vi "Temp_QCM_MKS_file.vi"() -> ()   [LabVIEW 2013]
doc: "This example demonstrates temperature control and monitoring.\n\nNote:\nBefore start this VI is it necessary:\n\n- preconfigure some specific parameters that are not supported by this driver (e.g. PV-I/O Type, Linearization type, Alarm Input Values... ) by Quick Codes, or by Eurotherm iTools or by instrument front panel controls\n- enter correct VISA Resource Descriptor, Device Address and Baud Rate into front-panel controls"
uses:
  LabVIEW Drivers for DVS instruments/_mks/common/mks pressure units.ctl
  LabVIEW Drivers for DVS instruments/_mks/common/mks status.ctl
  LabVIEW Drivers for DVS instruments/_mks/common/mks status control mode.ctl
  LabVIEW Drivers for DVS instruments/_mks/common/mks status learning mode.ctl
  LabVIEW Drivers for DVS instruments/_mks/common/mks status selection mode.ctl
  LabVIEW Drivers for DVS instruments/_mks/common/mks control direction.ctl
  LabVIEW Drivers for DVS instruments/_mks/common/mks setup communication mode.ctl
  LabVIEW Drivers for DVS instruments/_mks/common/mks setup termination character.ctl
  LabVIEW Drivers for DVS instruments/_mks/common/mks setpoint type.ctl
  LabVIEW Drivers for DVS instruments/_mks/common/mks control type.ctl
  <vilib>/Utility/file.llb/Write To Spreadsheet File (string).vi
  <instrlib>/Eurotherm 32xx Series/Eurotherm 32xx Series.lvlib
panel:
  in  "stop":bool
  in  "Tab Control":T1(tab)
  in  "Add comments to the data file here and click outside the comment box to submit.\nThe time at which comments are submitted is saved in the data file.":string
  out "New ALARM !":bool
  in  "Acknowledge All Alarms":bool
  in  "Controller  Mode":u8(ring) items=["Auto", "Manual"]
  in  "Temp Setpoint (C)":i16(slide)=25 min=0 max=1300 scale=0.0..500.0
  out "Temperature (C)":sgl
  out "Process Value - Chart":sgl(graph)
  in  "Keylock":u8(ring) items=["None", "All", "Edit", "mod", "mAn", "Stby", "tmr"]
  out "Alarm Output":bool
  in  "Alarm \nNumber (1)":u16=1 min=1 max=4
  out "Freq and Resistance Graph":T2(graph)
  out "pressure units 3":T3
  out "Waveform Chart 2":dbl(graph)
  out "status 2":T4
  out "Pressure 2":dbl
  in  "Control direction 3":T8
  in  "Setpoint 2":dbl(knob) min=0.0 max=100.0 scale=0.0..100.0
  out "Control direction 4":T8
  # "Configuring Instrument\n \nPlease Wait......\n\nChart will update in 20 sec"
  # "Instructions:\n\nMake sure all instruments are plugged into the correct ports, the correct port numbers are set, and all instruments are turned on. \n\nTo begin, click the RUN arrow on the toolbar, and wait 20 seconds for instruments to begin recording.\n\nTo end, click \"END DATA LOGGING\". DO NOT press the STOP button on the toolbar."
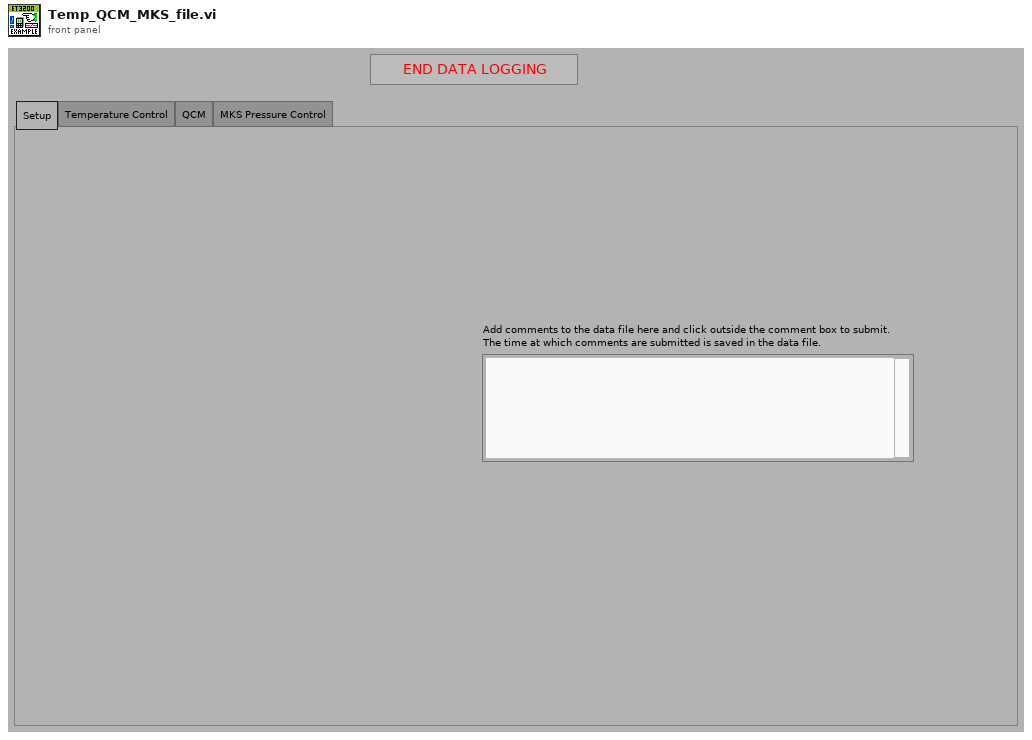
[diagram p1: front panel]
types:
  T1 = enum32{"Setup", "Temperature Control", "QCM", "MKS Pressure Control"}
  T2 = cluster{"XY chart data":cluster{"x":dbl, "y":dbl}[]}[]
  T3 = typedef "mks pressure units.ctl" = enum16{"Torr", "mTorr", "mbar", "ubar", "kPa", "Pa", "cmH2O", "inH2O"}
  T4 = typedef "mks status.ctl" = cluster{"control mode":T5, "learning mode":T6, "selection mode":T7}
  T5 = typedef "mks status control mode.ctl" = enum16{"local", "remote"}
  T6 = typedef "mks status learning mode.ctl" = enum16{"not learning", "learning system", "learning valve"}
  T7 = typedef "mks status selection mode.ctl" = enum16{"open", "close", "stop", "setpoint A", "setpoint B", "setpoint C", "setpoint D", "setpoint E", "analog setpoint"}
  T8 = typedef "mks control direction.ctl" = enum16{"direct", "reverse"}
  T9 = typedef "mks setup termination character.ctl" = enum16{"CRLF", "CR"}
  T10 = typedef "mks setup communication mode.ctl" = enum16{"8 databits no parity", "7 databits even parity"}
  T11 = typedef "mks control type.ctl" = enum16{"Self-Tuning", "PID"}
  T12 = typedef "mks setpoint type.ctl" = enum16{"position", "pressure"}
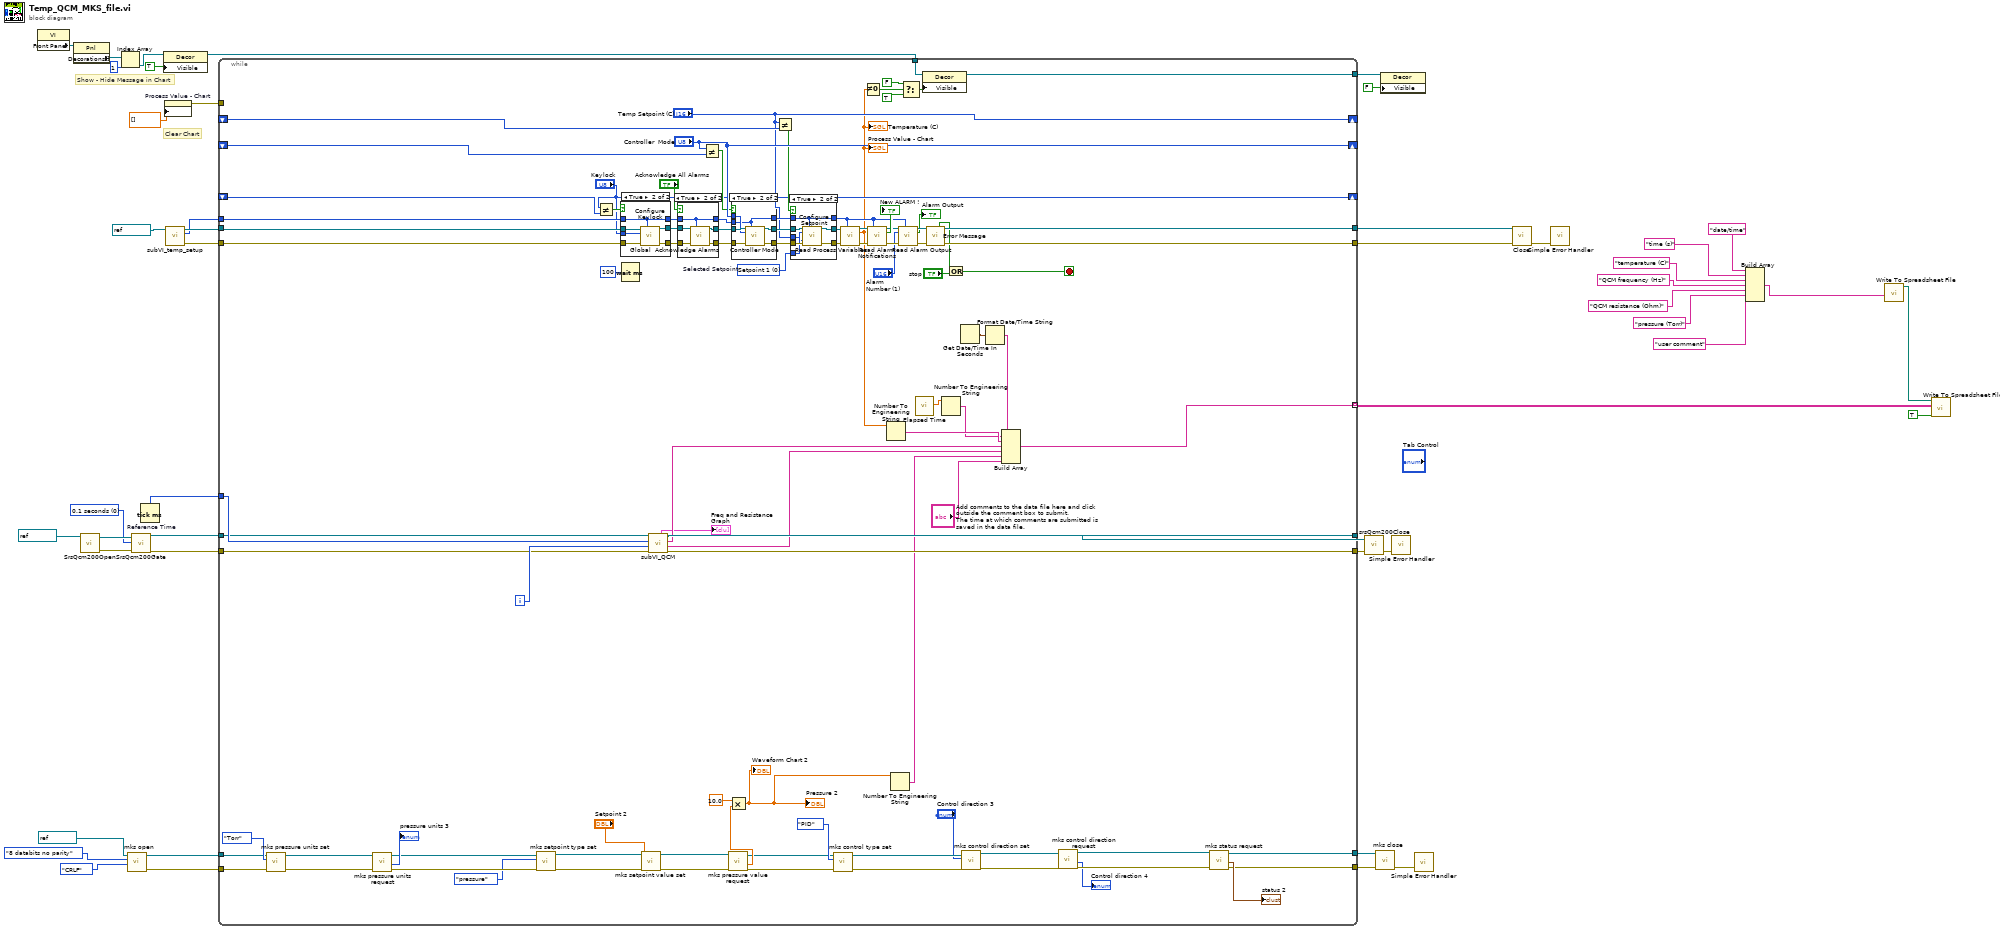
[diagram p0: block diagram]
diagram:
  w21 = u16 0 items=["0.1 seconds", "1.0 seconds", "10.0 seconds"] ("Gate in")
  # "Show - Hide Message in Chart"
  # "Clear Chart"
  n1 = property class="VI"() -> ("Front Panel"=w39:refnum<vi>)  [unwired: 2 in, 2 out]
  n2 = property class="Pnl"(reference=w39) -> ("Decorations[]"=w40:refnum<vi>[])  [unwired: 1 in, 2 out]
  n3 = call <instrlib>:"SrsQcm200Open.vi"("VISA in"=refnum<visa-resource-name> "COM6") -> ("error out"=w25:errorcluster, "VISA out"=w24:refnum<visa-resource-name>)  [unwired: 4 in]
  n4 = Index Array(array=w40, index=1) -> (element=w37:refnum<vi>)
  n5 = call "mks open.vi"("termination character"=mks_setup_termination_character."CRLF", "comm. mode"=mks_setup_communication_mode."8 databits no parity", "VISA in"=refnum<visa-resource-name> "COM5") -> ("error out"=w6:errorcluster, "VISA out"=w7:refnum<visa-resource-name>)  [unwired: 7 in]
  n6 = call <instrlib>:"SrsQcm200Gate.vi"("VISA in"=w24, "Gate in"=w21, "error in (no error)"=w25) -> ("VISA out"=w18:refnum<visa-resource-name>, "error out"=w17:errorcluster)  [unwired: 14 in, 1 out]
  n7 = Tick Count (ms) "Reference Time"() -> (millisecond timer value=w19:u32)
  n8 = property class="Decor"(reference=w37, "Visible"=TRUE) -> (reference out=w36:refnum<vi>)  [unwired: 1 in, 1 out]
  n9 = property on="Process Value - Chart" class="WFChart (strict)"("History Data"=sgl[] []) -> (error out=w32:errorcluster)  [unwired: 2 in, 1 out]
  n10 = call "subVI_temp_setup.vi"("VISA Refnum in"=refnum<visa-resource-name> "COM4" ("VISA resource name")) -> ("error out"=w45:errorcluster, "Unit Address (1)"=w26:u8, "VISA Refnum out"=w46:refnum<visa-resource-name>)  [unwired: 8 in]
  n11 = while {
    tunnel: w46 -> [w113]
    tunnel: w45 -> [w112]
    tunnel: w26 -> [w114]
    tunnel: [w134] -> w43
    tunnel: [w133] -> w44
    shift-right: ["Keylock"] -> _
    shift-left: _ -> [w123]
    shift-right: ["Controller  Mode"] -> _
    shift-left: _ -> [w120]
    shift-right: ["Temp Setpoint (C)"] -> _
    shift-left: _ -> [w118]
    tunnel: w36 -> [w98]
    tunnel: [w96] -> w34
    tunnel: w32 -> [_]
    tunnel: [w92] -> w20 mode=indexing
    tunnel: w19 -> [w90]
    tunnel: w18 -> [w89]
    tunnel: w17 -> [w88]
    tunnel: [w87] -> w16
    tunnel: [w86] -> w15
    tunnel: w7 -> [w56]
    tunnel: w6 -> [w55]
    tunnel: [w54] -> w4
    tunnel: [w53] -> w3
    i -> [w91]
    stop <- w127 stop-if-true
    w129 = u8 0 items=["Setpoint 1", "Setpoint 2", "Alternate Setpoint", "Target Setpoint"]  # Selected Setpoint
    n12 = call "mks pressure units set.vi"("error in (no error)"=w55, "pressure units"=mks_pressure_units."Torr", "VISA in"=w56) -> ("error out"=w69:errorcluster, "VISA out"=w68:refnum<visa-resource-name>)  [unwired: 7 in]
    n13 = call "mks pressure units request.vi"("error in (no error)"=w69, "VISA in"=w68) -> ("error out"=w71:errorcluster, "pressure units"=→"pressure units 3":T3, "VISA out"=w70:refnum<visa-resource-name>)  [unwired: 7 in]
    n14 = call "mks setpoint type set.vi"("error in (no error)"=w71, "setpoint type"=mks_setpoint_type."pressure", "VISA in"=w70) -> ("error out"=w59:errorcluster, "VISA out"=w58:refnum<visa-resource-name>)  [unwired: 7 in]
    n15 = Not Equal?(x="Keylock", y=w123) -> (x != y?=w122:bool)
    n16 = case shown="True" w122 {
      tunnel: w113 -> [w171 w178]
      tunnel: w112 -> [w170 w177]
      tunnel: [w171 w176] -> w142
      tunnel: [w170 w175] -> w141
      tunnel: w114 -> [w172 w174]
      tunnel: [w172 w174] -> w131
      tunnel: "Keylock" -> [_ w173]
      frame False {
      }
      frame True {
        n17 = call <instrlib>:"Configure Keylock.vi"("VISA resource name"=w178, "Unit Address (1)"=w174, "Keylock"=w173, "error in (no error)"=w177) -> ("VISA resource name out"=w176:refnum<visa-resource-name>, "error out"=w175:errorcluster)  [unwired: 10 in]
      }
    }
    n18 = Wait (ms)(milliseconds to wait=u32 100) -> ()  [unwired: 1 out]
    n19 = call "mks setpoint value set.vi"("error in (no error)"=w59, "setpoint"="Setpoint 2", "VISA in"=w58) -> ("error out"=w64:errorcluster, "VISA out"=w63:refnum<visa-resource-name>)  [unwired: 7 in]
    n20 = call "subVI_QCM.vi"("error in (no error)"=w88, "Loop iteration number"=w91, "millisecond timer value"=w90, "VISA Refnum in"=w89) -> ("error out"=w86:errorcluster, "Resistance (Ohm)"=w84:string, "Freq (Hz)"=w85:string, "VISA Refnum out"=w87:refnum<visa-resource-name>, "Freq and Resistance Graph"=→"Freq and Resistance Graph":T2)  [unwired: 3 in]
    n21 = case shown="True" "Acknowledge All Alarms" {
      tunnel: w142 -> [w163 w169]
      tunnel: w141 -> [w162 w168]
      tunnel: [w163 w167] -> w136
      tunnel: [w162 w166] -> w135
      tunnel: w131 -> [w164 w165]
      tunnel: [w164 w165] -> w130
      frame False {
      }
      frame True {
        n22 = call <instrlib>:"Global  Acknowledge Alarms.vi"("VISA resource name"=w169, "Unit Address (1)"=w165, "error in (no error)"=w168) -> ("VISA resource name out"=w167:refnum<visa-resource-name>, "error out"=w166:errorcluster)  [unwired: 11 in]
      }
    }
    n23 = Not Equal?(x="Controller  Mode", y=w120) -> (x != y?=w119:bool)
    n24 = call "mks pressure value request.vi"("error in (no error)"=w64, "VISA in"=w63) -> ("error out"=w66:errorcluster, "pressure"=w81:dbl, "VISA out"=w65:refnum<visa-resource-name>)  [unwired: 7 in]
    n25 = Multiply(x=10.0, y=w81) -> (x*y=w52:dbl)
    "Pressure 2" <- w52
    "Waveform Chart 2" <- w52
    n26 = case shown="True" w119 {
      tunnel: [w153 w161] -> w140
      tunnel: [w154 w160] -> w137
      tunnel: w136 -> [w154 w159]
      tunnel: w135 -> [w153 w158]
      tunnel: w130 -> [w155 w156]
      tunnel: "Controller  Mode" -> [_ w157]
      tunnel: [w155 w156] -> w128
      frame False {
      }
      frame True {
        n27 = call <instrlib>:"Controller Mode.vi"("VISA resource name"=w159, "Unit Address (1)"=w156, "Controller Mode (0: Auto)"=w157, "error in (no error)"=w158) -> ("VISA resource name out"=w160:refnum<visa-resource-name>, "error out"=w161:errorcluster)  [unwired: 10 in]
      }
    }
    n28 = Not Equal?(x="Temp Setpoint (C)", y=w118) -> (x != y?=w116:bool)
    n29 = case shown="True" w116 {
      tunnel: w140 -> [w143 w152]
      tunnel: [w143 w151] -> w139
      tunnel: [w144 w150] -> w138
      tunnel: w137 -> [w144 w149]
      tunnel: w129 -> [_ w148]
      tunnel: w128 -> [w145 w147]
      tunnel: [w145 w147] -> w103
      tunnel: "Temp Setpoint (C)" -> [_ w146]
      frame False {
      }
      frame True {
        n30 = call <instrlib>:"Configure Setpoint.vi"("VISA resource name"=w149, "Unit Address (1)"=w147, "Setpoint (0: Setpoint 1)"=w148, "Setpoint Value (0)"=w146, "error in (no error)"=w152) -> ("VISA resource name out"=w150:refnum<visa-resource-name>, "error out"=w151:errorcluster)  [unwired: 9 in]
      }
    }
    n31 = call "mks control type set.vi"("error in (no error)"=w66, "control type"=mks_control_type."PID", "VISA in"=w65) -> ("error out"=w76:errorcluster, "VISA out"=w75:refnum<visa-resource-name>)  [unwired: 7 in]
    n32 = call <instrlib>:"Read Process Variables.vi"("VISA resource name"=w138, "Unit Address (1)"=w103, "error in (no error)"=w139) -> ("VISA resource name out"=w111:refnum<visa-resource-name>, "Process Value"=w94:sgl, "error out"=w110:errorcluster)  [unwired: 9 in, 1 out]
    "Temperature (C)" <- w94
    "Process Value - Chart" <- w94
    n33 = Not Equal To 0?(x=w94) -> (x != 0?=w99:bool)
    n34 = call <instrlib>:"Read Alarm Notifications.vi"("VISA resource name"=w111, "Unit Address (1)"=w103, "error in (no error)"=w110) -> ("VISA resource name out"=w107:refnum<visa-resource-name>, "New Alarm"=→"New ALARM !":bool, "error out"=w108:errorcluster)  [unwired: 10 in]
    n35 = Number To Engineering String(4:w94) -> (0:w93:string)  [unwired: 3 in]
    n36 = Number To Engineering String(4:w52) -> (0:w51:string)  [unwired: 3 in]
    n37 = call <instrlib>:"Read Alarm Output.vi"("VISA resource name"=w107, "Unit Address (1)"=w103, "Alarm Number (1)"="Alarm \nNumber (1)", "error in (no error)"=w108) -> ("VISA resource name out"=w106:refnum<visa-resource-name>, "Alarm Output"=→"Alarm Output":bool, "error out"=w105:errorcluster)  [unwired: 9 in]
    n38 = Select(t=FALSE ("Visible"), s=w99, f=TRUE ("Visible")) -> (s? t:f=w101:bool)
    n39 = call "Elapsed Time"() -> ("Elapsed Time (s)"=w47:dbl)  [unwired: 12 in, 7 out]
    n40 = property class="Decor"(reference=w98, "Visible"=w101) -> (reference out=w96:refnum<vi>)  [unwired: 1 in, 1 out]
    n41 = call <instrlib>:"Error Message.vi"("VISA resource name"=w106, "error in (no error)"=w105) -> ("Status"=w125:bool, "VISA resource name out"=w134:refnum<visa-resource-name>, "error out"=w133:errorcluster)  [unwired: 9 in, 2 out]
    n42 = Number To Engineering String(4:w47) -> (0:w48:string)  [unwired: 3 in]
    n43 = Or(x=w125, y="stop") -> (x .or. y?=w127:bool)
    n44 = Get Date/Time In Seconds() -> (seconds since 1Jan1904=w95:timestamp)
    n45 = call "mks control direction set.vi"("error in (no error)"=w76, "direction"="Control direction 3", "VISA in"=w75) -> ("error out"=w77:errorcluster, "VISA out"=w78:refnum<visa-resource-name>)  [unwired: 7 in]
    n46 = Format Date/Time String(seconds (now)=w95) -> (date/time string=w49:string)  [unwired: 2 in]
    n47 = Build Array(w49, w48, w93, w85, w84, w51, "Add comments to the data file here and click outside the comment box to submit.\nThe time at which comments are submitted is saved in the data file.") -> (w92:string[])
    n48 = call "mks control direction request.vi"("error in (no error)"=w77, "VISA in"=w78) -> ("error out"=w74:errorcluster, "direction"=→"Control direction 4":T8, "VISA out"=w73:refnum<visa-resource-name>)  [unwired: 7 in]
    n49 = call "mks status request.vi"("error in (no error)"=w74, "VISA in"=w73) -> ("error out"=w53:errorcluster, "status"=→"status 2":T4, "VISA out"=w54:refnum<visa-resource-name>)  [unwired: 7 in]
  }
  n50 = call <instrlib>:"srsQcm200Close.vi"("error in"=w15, "Visa in"=w16) -> ("error out"=w22:errorcluster)  [unwired: 3 in]
  n51 = call "mks close.vi"("error in (no error)"=w3, "VISA in"=w4) -> ("error out"=w5:errorcluster)  [unwired: 9 in]
  n52 = property class="Decor"(reference=w34, "Visible"=FALSE) -> ()  [unwired: 1 in, 2 out]
  n53 = call <vilib>:"Simple Error Handler.vi"("error in (no error)"=w22) -> ()  [unwired: 4 in, 5 out]
  n54 = call <vilib>:"Simple Error Handler.vi"("error in (no error)"=w5) -> ()  [unwired: 4 in, 5 out]
  n55 = call <instrlib>:"Close.vi"("VISA resource name"=w43, "error in (no error)"=w44) -> ("error out"=w42:errorcluster)  [unwired: 13 in]
  n56 = call <vilib>:"Simple Error Handler.vi"("error in (no error)"=w42) -> ()  [unwired: 4 in, 5 out]
  n57 = Build Array("date/time", "time (s)", "temperature (C)", "QCM frequency (Hz)", "QCM resistance (Ohm)" ("element"), "pressure (Torr)" ("element"), "user comment" ("element")) -> (w29:string[])
  n58 = call-poly <vilib>:"Write To Spreadsheet File.vi"("1D data"=w29) -> ("new file path (Not A Path if cancelled)"=w28:path)  [unwired: 7 in]
  n59 = call-poly <vilib>:"Write To Spreadsheet File.vi"("append to file? (new file:F)"=TRUE, "2D data"=w20, "file path (dialog if empty)"=w28) -> ()  [unwired: 5 in, 1 out]
